vi "VISA.Get Available Device Info with PID and VID Lookup.vi"(6 "PID":string, 7 "Exact Match":bool, 8 "error in":errorcluster, 9 "VID":string="28DE", 10 "Description Contains":string, 11 "Alias Contains":string="COM") -> (0 "error out":errorcluster, 2 "Best Match":T1, 3 "Devices":T1[](array[typedef]))   [LabVIEW 2018]
uses:
  VISA.Device Info.ctl
  <vilib>/Instr/_visa.llb/VISA Find Search Mode.ctl
panel:
  # "Get VISA Device Info"
  # "COM"
  # "USB Serial Device"
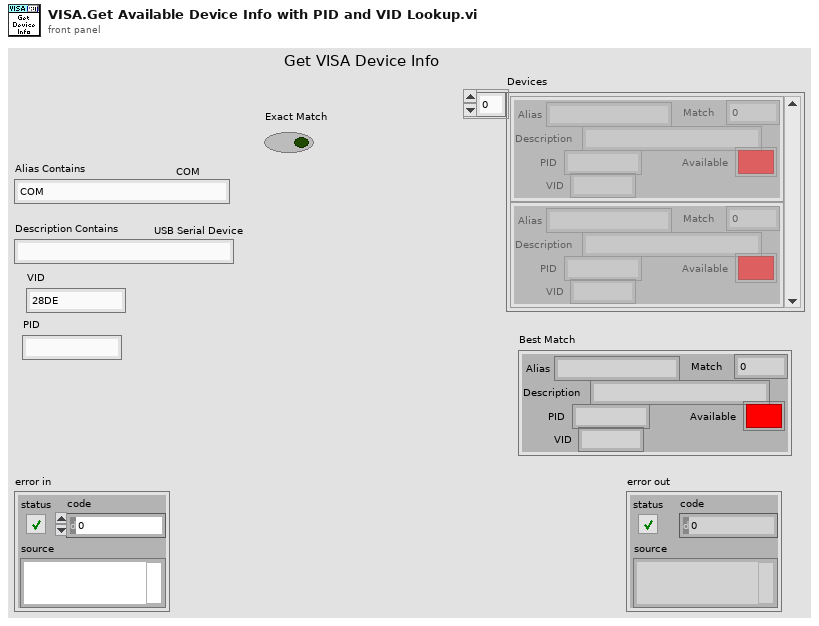
[diagram p1: front panel]
types:
  T1 = typedef "VISA.Device Info.ctl" = cluster{"Match":i32, "Alias":string, "Description":string, "Available":bool, "PID":string, "VID":string}
  T2 = typedef "VISA Find Search Mode.ctl" = u32
  T3 = cluster{"ID":string, "Type":string, "VID":string, "PID":string}[]
  T4 = cluster{"ID":string, "Type":string, "VID":string, "PID":string}
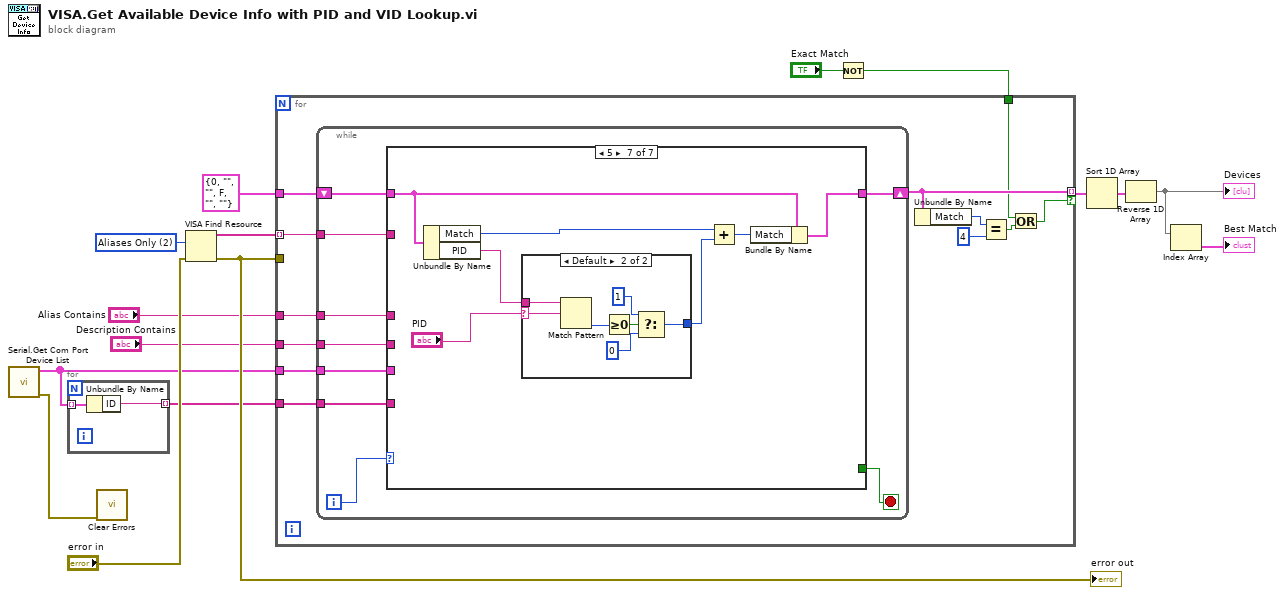
[diagram p0: block diagram]
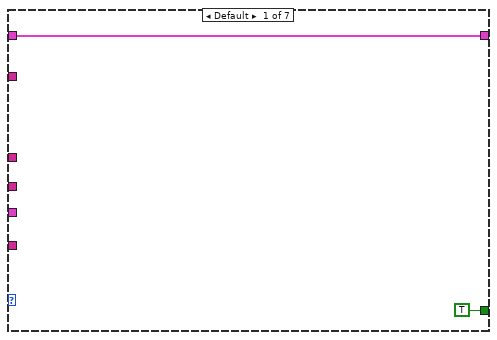
[diagram p2: hidden frame]
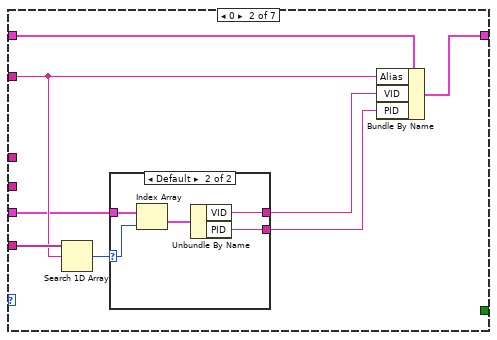
[diagram p3: hidden frame]
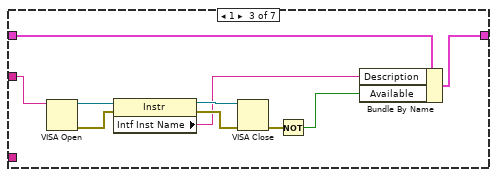
[diagram p5: hidden frame]
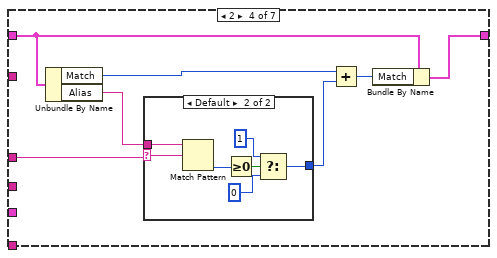
[diagram p6: hidden frame]
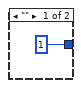
[diagram p7: hidden frame]
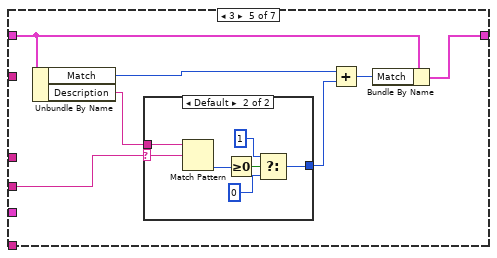
[diagram p8: hidden frame]
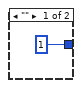
[diagram p9: hidden frame]
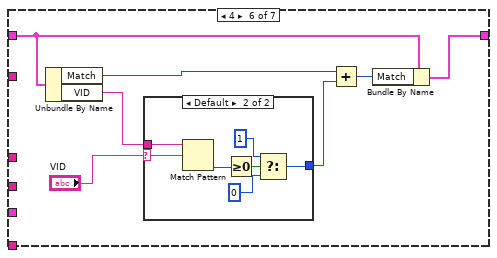
[diagram p10: hidden frame]
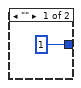
[diagram p11: hidden frame]
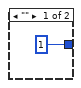
[diagram p12: hidden frame]
diagram:
  w16 = T2 2 items=["Canonical Names Only"=0, "Aliases Only"=2, "Include Matching Aliases"=3, "Include All Aliases"=4] ("Search Mode")
  n1 = call "Serial.Get Com Port Device List.vi"() -> ("error out"=w7:errorcluster, "Ports"=w6:T3)  [unwired: 10 in]
  n2 = for {
    tunnel: w6 -> [w18] mode=indexing
    tunnel: [w17] -> w5 mode=indexing
    n3 = Unbundle By Name(w18) -> ("ID"=w17:string)
  }
  n4 = call <vilib>:"Clear Errors.vi"("error in (no error)"=w7) -> ()  [unwired: 5 in, 2 out]
  n5 = VISA Find Resource(8:"error in", 10:w16) -> (0:w13:errorcluster, 3:w15:string[])  [unwired: 1 in, 1 out]
  "error out" <- w13
  n6 = Not(x="Exact Match") -> (.not. x?=w1:bool)
  n7 = for {
    tunnel: w15 -> [w29] mode=indexing
    tunnel: w13 -> [_]
    tunnel: [w24] -> w10 mode=indexing if=w19
    tunnel: "Alias Contains" -> [w28]
    tunnel: "Description Contains" -> [w27]
    tunnel: T1 {"Match"=0, "Alias"="", "Description"="", "Available"=FALSE, "PID"="", "VID"=""} ("Device Info") -> [w30]
    tunnel: w6 -> [w26]
    tunnel: w5 -> [w25]
    tunnel: w1 -> [w20]
    n8 = while {
      shift-right: [w32] -> w24
      shift-left: w30 -> [w39]
      tunnel: w29 -> [w37]
      tunnel: w28 -> [w36]
      tunnel: w27 -> [w35]
      tunnel: w26 -> [w34]
      tunnel: w25 -> [w33]
      i -> [w38]
      stop <- w31 stop-if-true
      n9 = case shown="5" w38 {
        tunnel: w39 -> [w41 w49 w64 w70 w85 w100 w115]
        tunnel: w37 -> [_ w47 w58 _ _ _ _]
        tunnel: w36 -> [_ _ _ w68 _ _ _]
        tunnel: w35 -> [_ _ _ _ w80 _ _]
        tunnel: w34 -> [_ w45 _ _ _ _ _]
        tunnel: w33 -> [_ w48 _ _ _ _ _]
        tunnel: [w41 w42 w63 w71 w86 w101 w116] -> w32
        tunnel: [TRUE _ _ _ _ _ _] -> w31
        frame Default {
        }
        frame 0 {
          n10 = Search 1D Array(1D array=w48, element=w47) -> (index of element=w46:i32)  [unwired: 1 in]
          n11 = case shown="Default" w46 {
            selector: w46 -> [_ w53]
            tunnel: w45 -> [_ w54]
            tunnel: [_ w51] -> w44
            tunnel: [_ w50] -> w43
            frame -1 {
            }
            frame Default {
              n12 = Index Array(array=w54, index=w53) -> (element=w52:T4)
              n13 = Unbundle By Name(w52) -> ("VID"=w51:string, "PID"=w50:string)
            }
          }
          n14 = Bundle By Name(cluster=w49, "Alias"=w47, "VID"=w44, "PID"=w43) -> (w42:T1)
        }
        frame 1 {
          n15 = VISA Open(VISA resource name=w58) -> (VISA resource name=w62:refnum<visa-resource-name>, error out=w59:errorcluster)  [unwired: 4 in]
          n16 = property class="Instr"(reference=w62, error in=w59) -> (reference out=w61:refnum<visa-resource-name>, error out=w60:errorcluster, "Intf Inst Name"=w57:string)
          n17 = VISA Close(VISA resource name=w61, error in (no error)=w60) -> (error out=w56:errorcluster)
          n18 = Not(x=w56) -> (.not. x?=w55:bool)
          n19 = Bundle By Name(cluster=w64, "Description"=w57, "Available"=w55) -> (w63:T1)
        }
        frame 2 {
          n20 = Unbundle By Name(w70) -> ("Match"=w67:i32, "Alias"=w69:string)
          n21 = case shown="Default" w68 {
            selector: w68 -> [_ w77]
            tunnel: w69 -> [_ w79]
            tunnel: [1 w73] -> w65
            frame "" {
            }
            frame Default {
              n22 = Match Pattern(string=w79, regular expression=w77) -> (offset past match=w78:i32)  [unwired: 1 in, 3 out]
              n23 = Greater Or Equal To 0?(x=w78) -> (x >= 0?=w76:bool)
              n24 = Select(t=1, s=w76, f=0) -> (s? t:f=w73:i32)
            }
          }
          n25 = Add(x=w67, y=w65) -> (x+y=w66:i32)
          n26 = Bundle By Name(cluster=w70, "Match"=w66) -> (w71:T1)
        }
        frame 3 {
          n27 = Unbundle By Name(w85) -> ("Match"=w83:i32, "Description"=w84:string)
          n28 = case shown="Default" w80 {
            selector: w80 -> [_ w92]
            tunnel: w84 -> [_ w94]
            tunnel: [1 w88] -> w81
            frame "" {
            }
            frame Default {
              n29 = Match Pattern(string=w94, regular expression=w92) -> (offset past match=w93:i32)  [unwired: 1 in, 3 out]
              n30 = Greater Or Equal To 0?(x=w93) -> (x >= 0?=w91:bool)
              n31 = Select(t=1, s=w91, f=0) -> (s? t:f=w88:i32)
            }
          }
          n32 = Add(x=w83, y=w81) -> (x+y=w82:i32)
          n33 = Bundle By Name(cluster=w85, "Match"=w82) -> (w86:T1)
        }
        frame 4 {
          n34 = Unbundle By Name(w100) -> ("Match"=w98:i32, "VID"=w99:string)
          n35 = case shown="Default" "VID" {
            selector: "VID" -> [_ w107]
            tunnel: w99 -> [_ w109]
            tunnel: [1 w103] -> w96
            frame "" {
            }
            frame Default {
              n36 = Match Pattern(string=w109, regular expression=w107) -> (offset past match=w108:i32)  [unwired: 1 in, 3 out]
              n37 = Greater Or Equal To 0?(x=w108) -> (x >= 0?=w106:bool)
              n38 = Select(t=1, s=w106, f=0) -> (s? t:f=w103:i32)
            }
          }
          n39 = Add(x=w98, y=w96) -> (x+y=w97:i32)
          n40 = Bundle By Name(cluster=w100, "Match"=w97) -> (w101:T1)
        }
        frame 5 {
          n41 = Unbundle By Name(w115) -> ("Match"=w113:i32, "PID"=w114:string)
          n42 = case shown="Default" "PID" {
            selector: "PID" -> [_ w122]
            tunnel: w114 -> [_ w124]
            tunnel: [1 w118] -> w111
            frame "" {
            }
            frame Default {
              n43 = Match Pattern(string=w124, regular expression=w122) -> (offset past match=w123:i32)  [unwired: 1 in, 3 out]
              n44 = Greater Or Equal To 0?(x=w123) -> (x >= 0?=w121:bool)
              n45 = Select(t=1, s=w121, f=0) -> (s? t:f=w118:i32)
            }
          }
          n46 = Add(x=w113, y=w111) -> (x+y=w112:i32)
          n47 = Bundle By Name(cluster=w115, "Match"=w112) -> (w116:T1)
        }
      }
    }
    n48 = Unbundle By Name(w24) -> ("Match"=w23:i32)
    n49 = Equal?(x=w23, y=4) -> (x = y?=w21:bool)
    n50 = Or(x=w20, y=w21) -> (x .or. y?=w19:bool)
  }
  n51 = Sort 1D Array(array=w10) -> (sorted array=w9:T1[])
  n52 = Reverse 1D Array(array=w9) -> (reversed array=w4:T1[])
  "Devices" <- w4
  n53 = Index Array(array=w4) -> (element=→"Best Match":T1)  [unwired: 1 in]
